vi "Airmar Read Sensor Data.vi"(8 "error (in)":errorcluster, 9 "NotifierReff":T1 caption="NotifierReff 2", 11 "VISA resource name (in)":refnum<visa-resource-name>="COM1") -> (0 "error (out)":errorcluster, 3 "VISA resource name (out)":refnum<visa-resource-name>)   [LabVIEW 2013]
doc: "This VI reads one sentence of data from the serial port associated with the WeatherStation Sensor (which must have been initialized previously using the \"1A Helper - Init Sensor.vi\"). \n\nIt reads one byte at a time, first waiting for the \"$\" (indicating the start of a sentence), then saving all bytes until a \"*ss\" is reached (the checksum, indicating the end of a sentence)."
uses:
  Data/TypeDefs/Notifiers.ctl
  Data/TypeDefs/UTM Location.ctl
  Data/TypeDefs/GPS Sensor Status.ctl
  Data/TypeDefs/Sail Set Suggestions.ctl
  Data/TypeDefs/Rudder Set Suggestions.ctl
panel:
  out "NMEA sentence":string
  out "Current Status":enum16{"Waiting", "Reading", "Time Out!"}(ring)
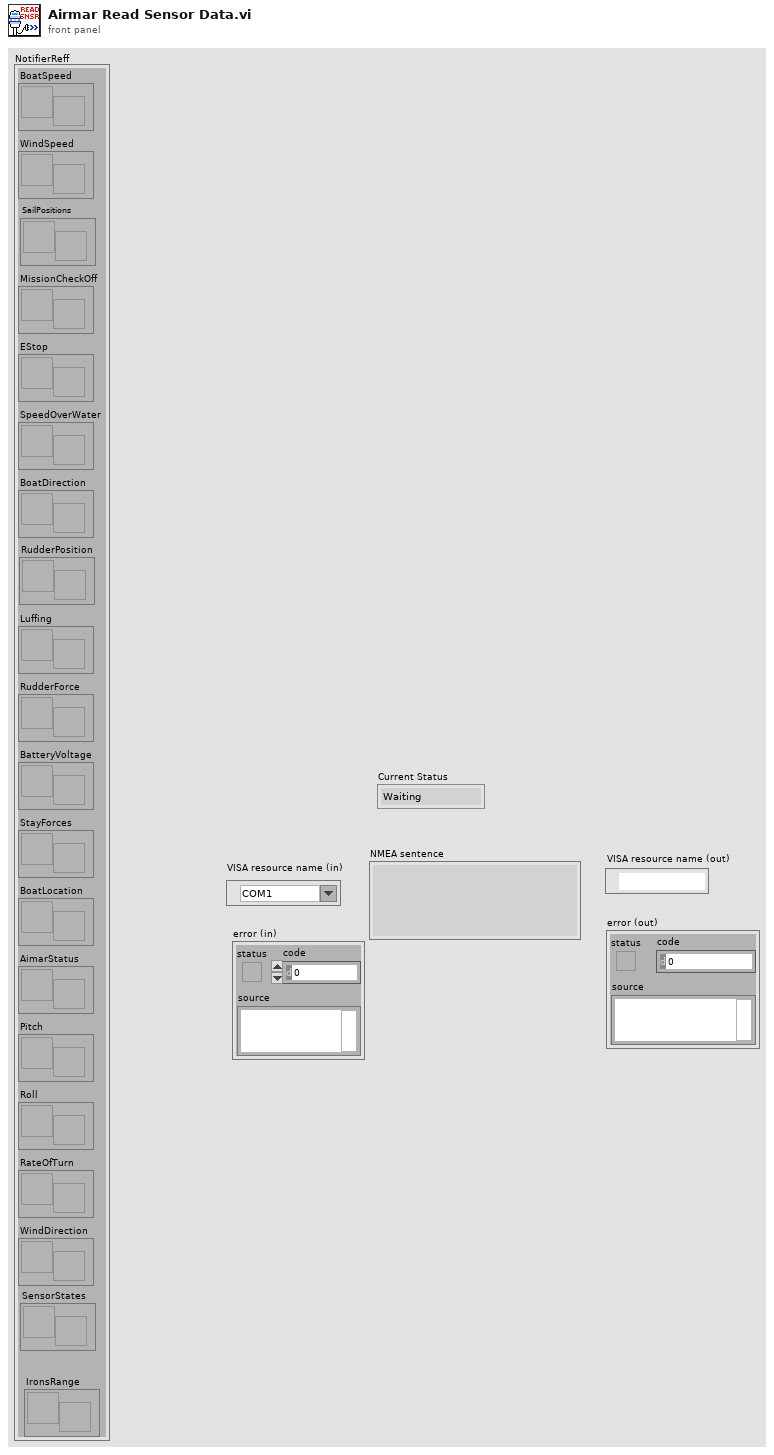
[diagram p1: front panel]
types:
  T1 = typedef "Notifiers.ctl" = cluster{"BoatSpeed":refnum<notifier>, "WindSpeed":refnum<notifier>, "MissionCheckOff":refnum<notifier>, "EStop":refnum<notifier>, "SpeedOverWater":refnum<notifier>, "BoatDirection":refnum<notifier>, "Luffing":refnum<notifier>, "RudderForce":refnum<notifier>, "BatteryVoltage":refnum<notifier>, "StayForces":refnum<notifier>, "BoatLocation":refnum<notifier>, "AimarStatus":refnum<notifier>, "Pitch":refnum<notifier>, "Roll":refnum<notifier>, "RateOfTurn":refnum<notifier>, "WindDirection":refnum<notifier>, "SailPositions":refnum<notifier>, "RudderPosition":refnum<notifier>, "SensorStates":refnum<notifier>, "IronsRange":refnum<notifier>}
  T2 = typedef "GPS Sensor Status.ctl" = cluster{"Sensor Connected":bool, "Sensor OK":bool, "GPS Lock":bool, "Sensor Initialized":bool}
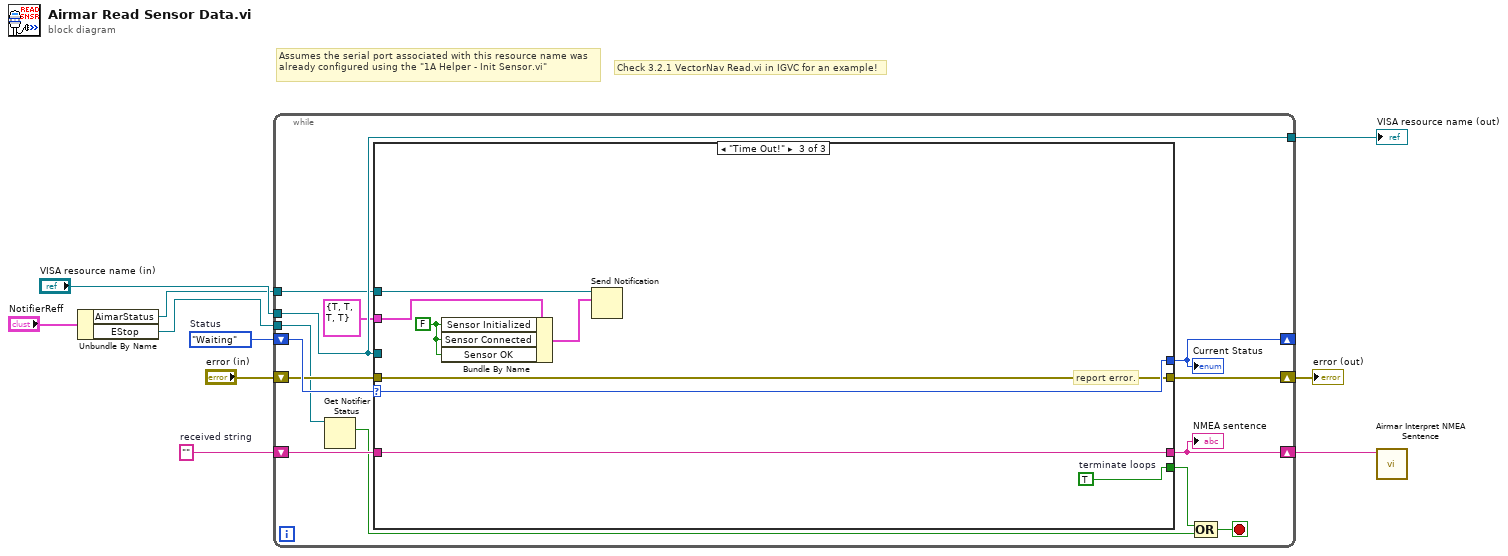
[diagram p0: block diagram]
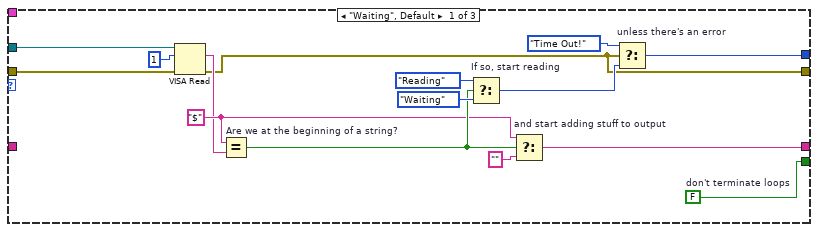
[diagram p2: hidden frame]
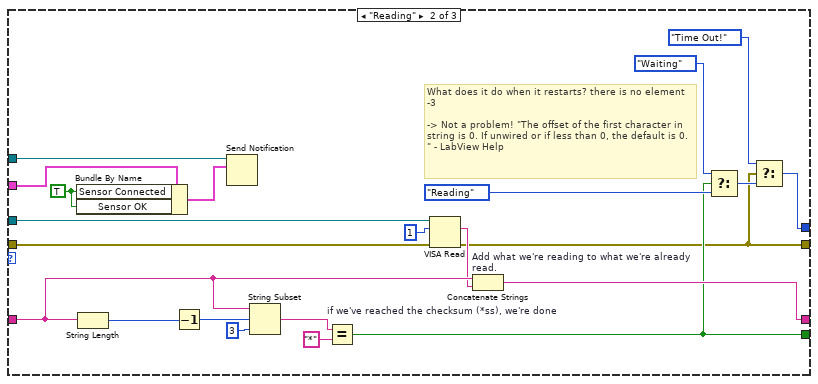
[diagram p3: hidden frame]
diagram:
  w7 = enum16{"Waiting", "Reading", "Time Out!"}."Waiting"  # Status
  w8 = ""  # received string
  # "Assumes the serial port associated with this resource name was already configured using the \"1A Helper - Init Sensor.vi\""
  # "Check 3.2.1 VectorNav Read.vi in IGVC for an example!"
  n1 = Unbundle By Name("NotifierReff") -> ("AimarStatus"=w1:refnum<notifier>, "EStop"=w2:refnum<notifier>)
  n2 = while {
    shift-right: [w16] -> w4
    shift-left: w8 -> [w23]
    shift-right: [w20] -> _
    shift-left: w7 -> [w22]
    tunnel: "VISA resource name (in)" -> [w15]
    shift-right: [w18] -> w5
    shift-left: "error (in)" -> [w19]
    tunnel: [w15] -> w6
    tunnel: w2 -> [w13]
    tunnel: w1 -> [w12]
    stop <- w21 stop-if-true
    n3 = Get Notifier Status(notifier=w13) -> (current notification=w14:bool)  [unwired: 1 in, 4 out]
    n4 = case shown="\"Time Out!\"" w22 {
      selector: w22 -> [_ _ w68]
      tunnel: w23 -> [_ w54 w67]
      tunnel: [w24 w60 w67] -> w16
      tunnel: [w29 w47 w68] -> w20
      tunnel: w15 -> [w32 w50 _]
      tunnel: w19 -> [w30 w48 w65]
      tunnel: [w27 w43 w65] -> w18
      tunnel: [w25 w44 w66] -> w17
      tunnel: w12 -> [_ w42 w62]
      tunnel: T2 {"Sensor Connected"=TRUE, "Sensor OK"=TRUE, "GPS Lock"=TRUE, "Sensor Initialized"=TRUE} ("input cluster") -> [_ w41 w64]
      frame "Waiting", Default {
        w25 = FALSE  # don't terminate loops
        w34 = "$" ("x")
        n5 = VISA Read(VISA resource name=w32, byte count=u32 1, error in (no error)=w30) -> (read buffer=w33:string, error out=w27:errorcluster)  [unwired: 2 out]
        n6 = Equal? "Are we at the beginning of a string?"(x=w34, y=w33) -> (x = y?=w35:bool)
        n7 = Select "If so, start reading"(t=enum16{"Waiting", "Reading", "Time Out!"}."Reading", s=w35, f=enum16{"Waiting", "Reading", "Time Out!"}."Waiting" ("Current Status")) -> (s? t:f=w28:enum16{"Waiting", "Reading", "Time Out!"})
        n8 = Select "and start adding stuff to output"(t=w34, s=w35, f="") -> (s? t:f=w24:string)
        n9 = Select "unless there's an error"(t=enum16{"Waiting", "Reading", "Time Out!"}."Time Out!", s=w27, f=w28) -> (s? t:f=w29:enum16{"Waiting", "Reading", "Time Out!"})
      }
      frame "Reading" {
        w39 = TRUE ("Sensor Connected")
        # "What does it do when it restarts? there is no element -3\n\n-> Not a problem! \"The offset of the first character in string is 0. If unwired or if less than 0, the default is 0. \" - LabView Help"
        n10 = Bundle By Name(cluster=w41, "Sensor Connected"=w39, "Sensor OK"=w39) -> (w40:T2)
        n11 = String Length(string=w54) -> (length=w59:i32)
        n12 = Decrement(x=w59) -> (x-1=w58:i32)
        n13 = Send Notification(notification=w40, notifier=w42) -> ()  [unwired: 1 in, 2 out]
        n14 = String Subset(string=w54, offset (0)=w58, length (rest)=3 ("length (rest)")) -> (substring=w56:string)
        n15 = Equal? "if we've reached the checksum (*ss), we're done"(x=w56, y="*") -> (x = y?=w44:bool)
        n16 = VISA Read(VISA resource name=w50, byte count=u32 1, error in (no error)=w48) -> (read buffer=w53:string, error out=w43:errorcluster)  [unwired: 2 out]
        n17 = Concatenate Strings "Add what we're reading to what we're already read."(w54, w53) -> (w60:string)
        n18 = Select(t=enum16{"Waiting", "Reading", "Time Out!"}."Waiting", s=w44, f=enum16{"Waiting", "Reading", "Time Out!"}."Reading" ("Status")) -> (s? t:f=w46:enum16{"Waiting", "Reading", "Time Out!"})
        n19 = Select(t=enum16{"Waiting", "Reading", "Time Out!"}."Time Out!", s=w43, f=w46) -> (s? t:f=w47:enum16{"Waiting", "Reading", "Time Out!"})
      }
      frame "Time Out!" {
        w61 = FALSE ("Sensor Initialized")
        w66 = TRUE  # terminate loops
        # "report error."
        n20 = Bundle By Name(cluster=w64, "Sensor Initialized"=w61, "Sensor Connected"=w61, "Sensor OK"=w61) -> (w63:T2)
        n21 = Send Notification(notification=w63, notifier=w62) -> ()  [unwired: 1 in, 2 out]
      }
    }
    "Current Status" <- w20
    "NMEA sentence" <- w16
    n22 = Compound Arithmetic op=OR(w17, w14) -> (w21:bool)
  }
  "VISA resource name (out)" <- w6
  "error (out)" <- w5
  n23 = call "Airmar Interpret NMEA Sentence.vi"("NMEA Sentence"=w4) -> ()  [unwired: 11 in]
